vi "TREE_Set Node Open or Close__jki_lib_tree_control -- VI Tester.vi"(8 "error in (no error)":errorcluster, 9 "Open (F)":bool, 10 "Tag":string, 11 "Tree Reference In":refnum<vi>) -> (0 "error out":errorcluster, 2 "Tag Dup":string, 3 "Tree Reference Out":refnum<vi>)   [LabVIEW 2011]
panel:
  # "Copyright © 2008 James Kring, Inc. All rights reserved.\n\nAuthor: Philippe Guerit [philippe.guerit@jameskring.com]\n             [alternate email: PJM_LabVIEW@yahoo.com]\n\nThis library is provided \"AS IS\" ,WITHOUT WARRANTIES OR \nCONDITIONS OF ANY KIND, either express or implied.\n\nJames Kring, Inc. -- http://www.jameskring.com"
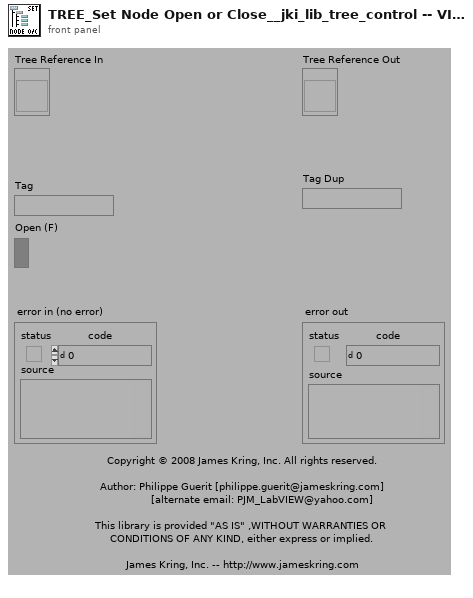
[diagram p1: front panel]
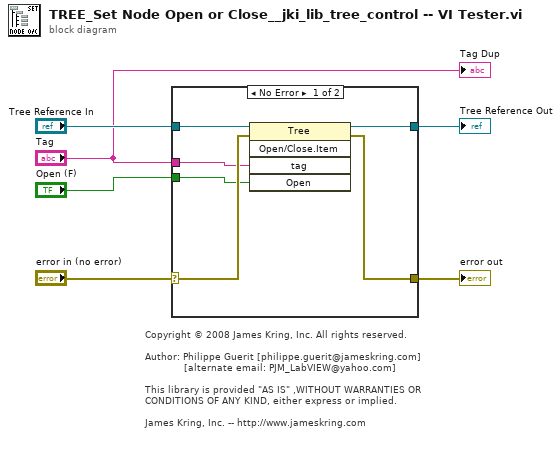
[diagram p0: block diagram]
diagram:
  # "Copyright © 2008 James Kring, Inc. All rights reserved.\n\nAuthor: Philippe Guerit [philippe.guerit@jameskring.com]\n             [alternate email: PJM_LabVIEW@yahoo.com]\n\nThis library is provided \"AS IS\" ,WITHOUT WARRANTIES OR \nCONDITIONS OF ANY KIND, either express or implied.\n\nJames Kring, Inc. -- http://www.jameskring.com"
  n1 = case shown="No Error" "error in (no error)" {
    selector: "error in (no error)" -> [w10 w14]
    tunnel: "Tree Reference In" -> [w12 w13]
    tunnel: [w11 w13] -> w5
    tunnel: [w9 w14] -> w3
    tunnel: "Tag" -> [w8 _]
    tunnel: "Open (F)" -> [w7 _]
    frame No Error {
      n2 = invoke class="Tree" method="Open/Close.Item"(reference=w12, error in=w10, "tag"=w8, "Open"=w7) -> (reference out=w11:refnum<vi>, error out=w9:errorcluster)  [unwired: 1 in, 3 out]
    }
    frame Error {
    }
  }
  "Tree Reference Out" <- w5
  "error out" <- w3
  "Tag Dup" <- "Tag"
